vi "RSNRPZ Set Sync Port.vi"(8 "error in (no error)":errorcluster, 9 "Port (IO Signal)":u32(ring)=1 items=["IO Signal"=1, "TRIG2 IO Signal"=5], 10 "Channel (1)":i32=1, 11 "VISA session":refnum<visa-resource-name> caption="VISA resource name") -> (0 "error out":errorcluster, 3 "dup VISA session":refnum<visa-resource-name> caption="VISA resource name")   [LabVIEW 2010]
doc: "This VI sets the sync port.\n\nRemote-control command(s):\nTRIG:SYNC:PORT"
uses:
  rsnrpz_32.dll
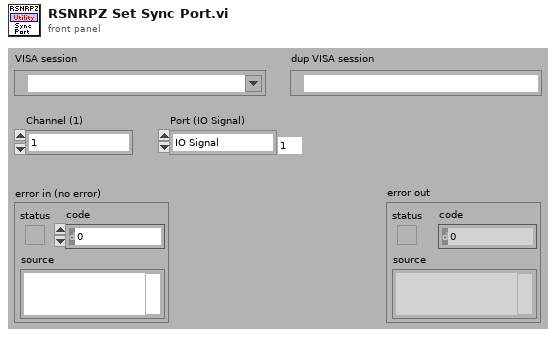
[diagram p1: front panel]
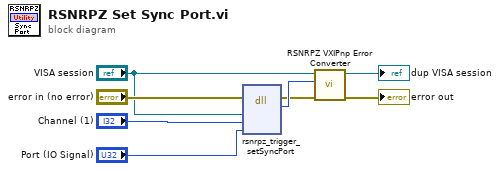
[diagram p0: block diagram]
diagram:
  n1 = dll-call lib="rsnrpz_32.dll" fn="rsnrpz_trigger_setSyncPort"(error in="error in (no error)", "Instrument Handle"="VISA session", "Channel"="Channel (1)", "Port"="Port (IO Signal)") -> (error out=w5:errorcluster, w6:i32)  [unwired: 5 in, 1 out]
  n2 = call <instrlib>:"RSNRPZ VXIPnp Error Converter.vi"("error in"=w5, "VXIPnp error code"=w6, "VISA session"="VISA session") -> ("error out"=→"error out":errorcluster, "dup VISA session"=→"dup VISA session":refnum<visa-resource-name>)  [unwired: 7 in]
